vi "blfind_EChemDev.vi"(6 "error in (no error)":errorcluster, 9 "DLL Path":path) -> (0 "error out":errorcluster, 3 "device table":string[][](array[string]))   [LabVIEW 2022 SP3, in "EClib functions.lvlib"]
uses:
  EClib functions.lvlib
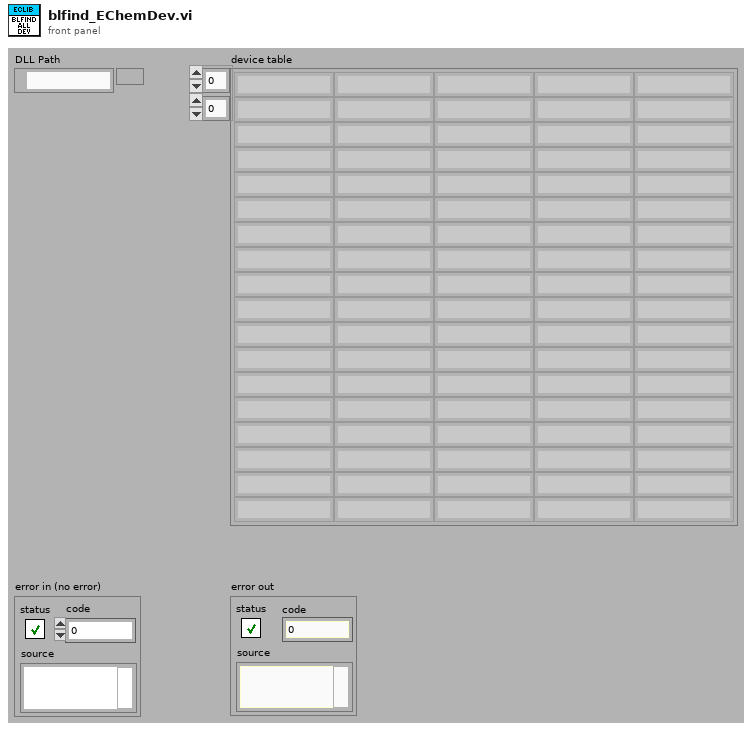
[diagram p1: front panel]
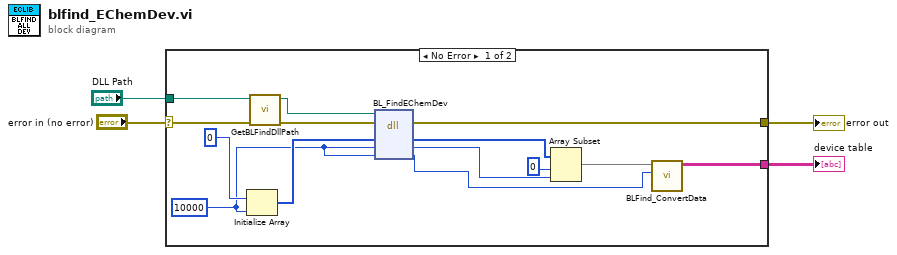
[diagram p0: block diagram]
diagram:
  n1 = case shown="No Error" "error in (no error)" {
    selector: "error in (no error)" -> [w9 w19]
    tunnel: [w6 w19] -> w3
    tunnel: [w10 _] -> w2
    tunnel: "DLL Path" -> [w5 _]
    frame No Error {
      w16 = 10000 ("dimension size")
      n2 = Initialize Array(u8 0, w16) -> (w17:u8[])
      n3 = call "GetBLFindDllPath.vi"("error in (no error)"=w9, "DLL Path"=w5) -> ("error out"=w8:errorcluster, "BlfindDLLPath"=w7:path)  [unwired: 8 in]
      n4 = dll-call lib="C:/EC-Lab Development Package/lib/blfind.dll" fn="BL_FindEChemDev"(path in=w7, error in=w8, "pLstdev"=w17, "psize"=w16, "pNbrDev"=w16) -> (error out=w6:errorcluster, "pLstdev"=w14:u16[], "psize"=w13:u32, "pNbrDev"=w12:u32)  [unwired: 2 in, 1 out]
      n5 = Array Subset(array=w14, index=0, length=w13) -> (w11:u16[])
      n6 = call "BLFind_ConvertData.vi"("pNbrDev"=w12, "pLstdev"=w11) -> ("device table"=w10:string[][])  [unwired: 9 in]
    }
    frame Error {
    }
  }
  "error out" <- w3
  "device table" <- w2
